vi "Durability_will_2012_07_04.vi"() -> ()   [LabVIEW 2011]
uses:
  <vilib>/DAQmx/write.llb/DAQmx Write (Counter Time 1Chan 1Samp).vi
  <vilib>/DAQmx/read.llb/DAQmx Read (Analog 1D Wfm NChan NSamp).vi
  <vilib>/express/express shared/ex_Modify Signal Name.vi
  <vilib>/measure/madcrms.llb/Basic Averaged DC-RMS for 1 Chan.vi
  <vilib>/DAQmx/miscellaneous.llb/DAQmx Fill In Error Info.vi
  <vilib>/express/express arith-compare/Formula/XNode/ExpressFormulaBlockNode.xnode
  <vilib>/measure/NI_MAPro.lvlib
  <vilib>/Analysis/NI_AALBase.lvlib
panel:
  out "Collected Signals":dynamicdata(graph)
  out "Table":string[][](table)
  in  "Filename 2":path=path "\\\\vmware-host\\Shared Folders/Desktop/long.tdms" caption="Filename"
  in  "Filename":path=path "\\\\vmware-host\\Shared Folders/Desktop/short.tdms"
  out "RPM Graph":dbl(graph)
  out "Motor RPM":dbl format="%#.0f"
  out "Motor Power (watts)":dbl format="%#.4f"
  out "Power to MC1 (watts)":dbl format="%#.4f"
  out "Voltage to MC1 (volts)":dbl format="%#.4f"
  out "Current to MC1  (amps)":dbl format="%#.4f"
  in  "Manual Start":bool
  in  "Power \nSetting":i8(slide) min=0 max=100 step=10 scale=0.0..100.0
  out "Power Setting (%)":dbl format="%#.2f"
  out "Motor Temp (F)":dbl format="%.1f"
  out "Tank Temp (F)":dbl format="%.1f"
  in  "Quit 4":bool
  out "Motor Power Over Time":dbl(graph)
  out "Phase to Phase Voltage":waveform(dbl)(graph)
  out "Phase Current":waveform(dbl)(graph)
  # "Motor Power and RPM"
  # "Temperature"
  # "MC1"
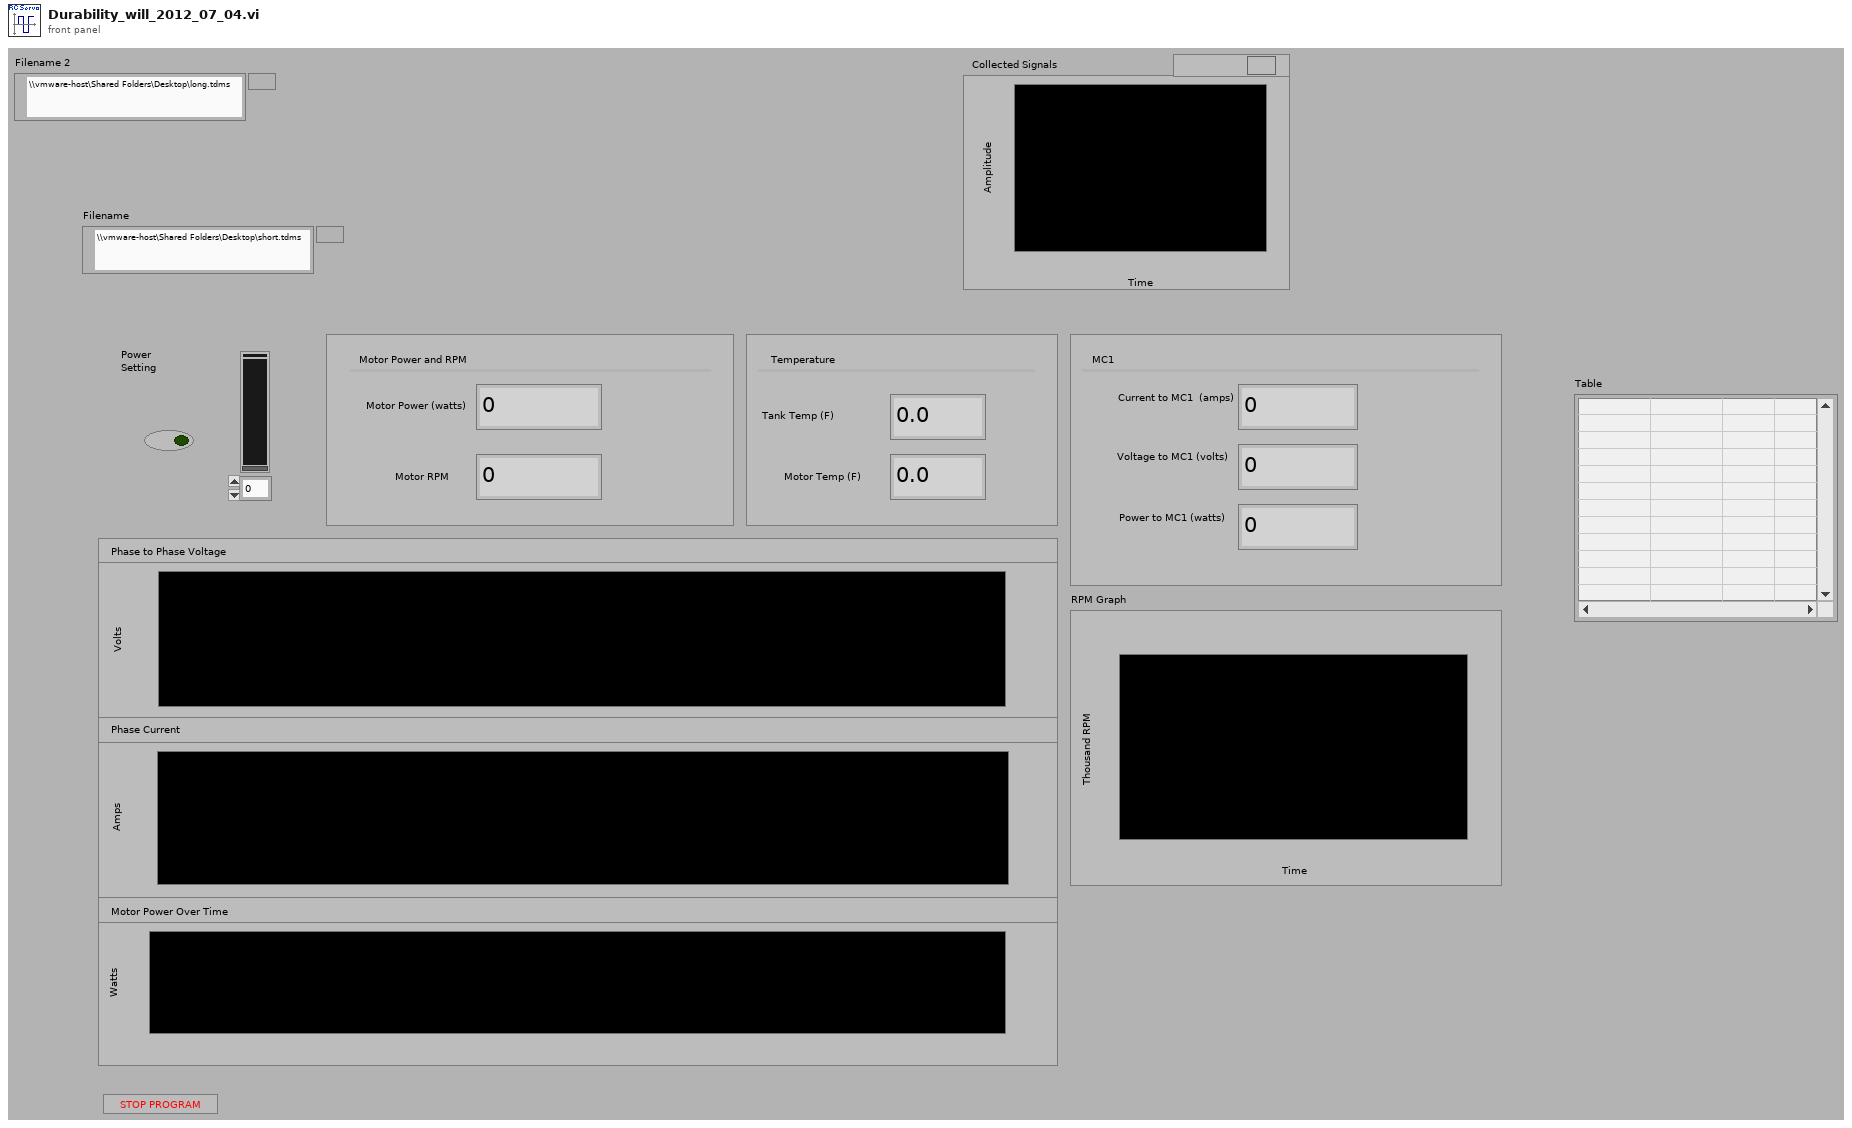
[diagram p1: front panel]
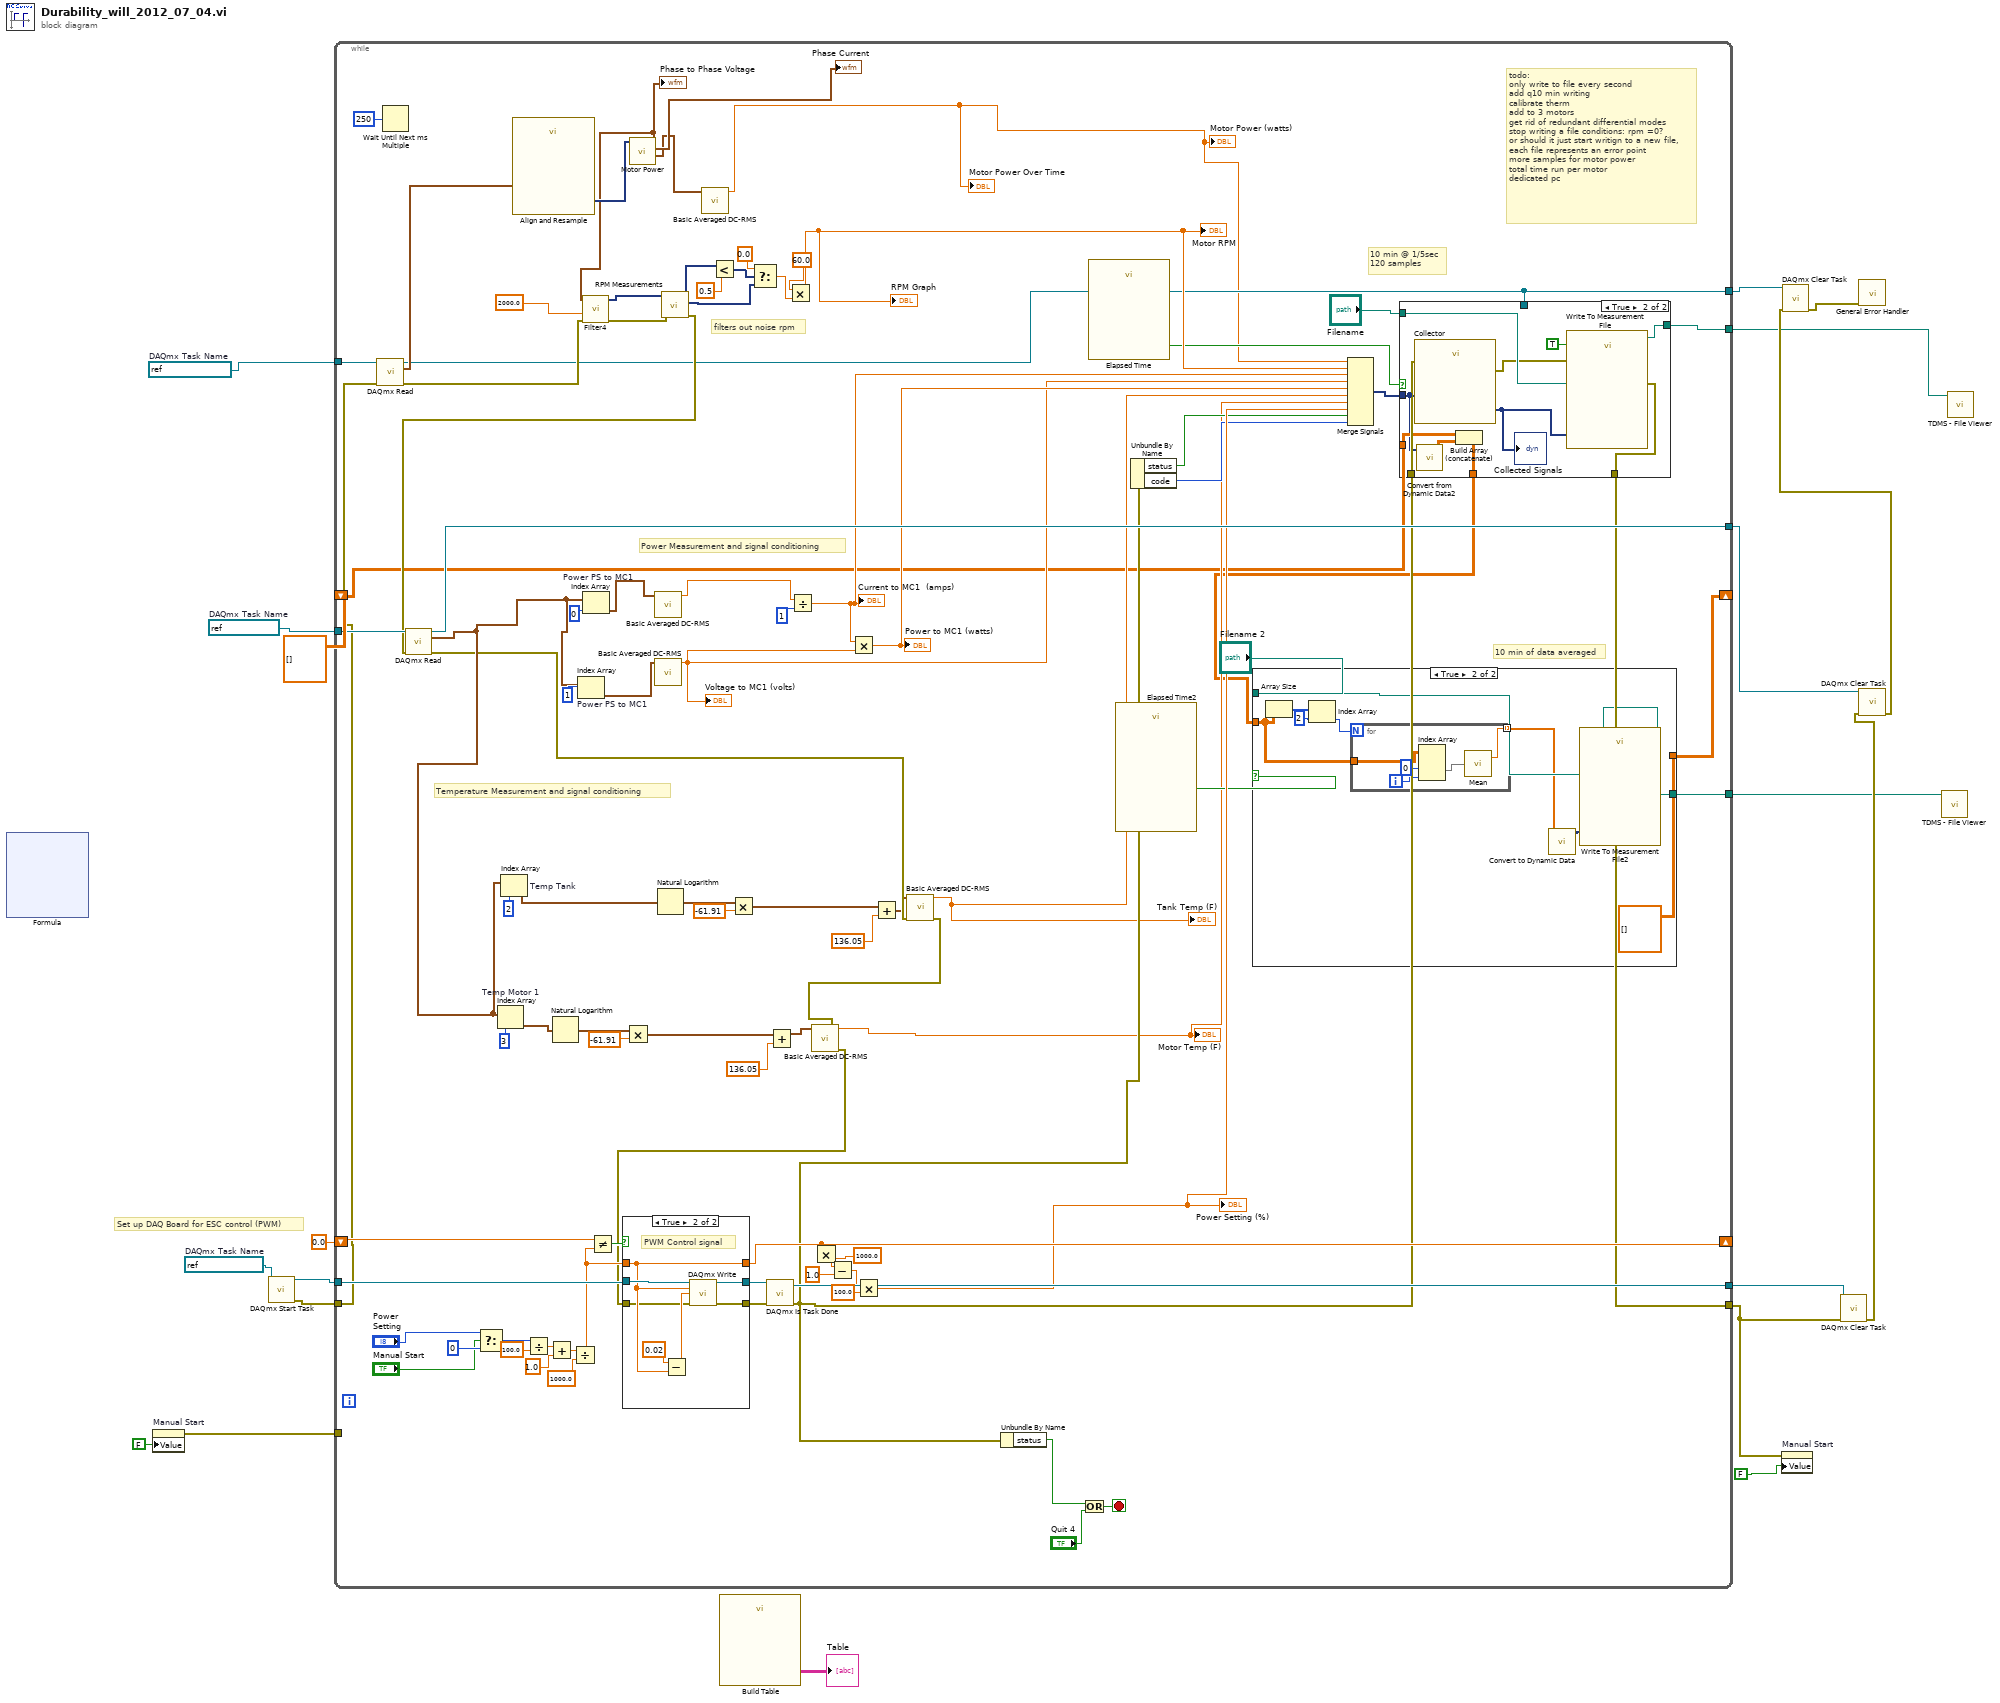
[diagram p0: block diagram]
diagram:
  w11 = refnum<k21> "PWM Signal"  # DAQmx Task Name
  w16 = refnum<k21> "MC Power"  # DAQmx Task Name
  w17 = refnum<k21> "Motor Power"  # DAQmx Task Name
  # "Set up DAQ Board for ESC control (PWM)"
  n1 = xnode "Formula"() -> ()  [unwired: 2 in, 2 out]
  n2 = property on="Manual Start" class="Bool (strict)"("Value"=FALSE ("Run Motor")) -> (error out=w14:errorcluster)  [unwired: 2 in, 1 out]
  n3 = call <vilib>:"DAQmx Start Task.vi"("task/channels in"=w11) -> ("task out"=w10:refnum<k21>, "error out"=w9:errorcluster)  [unwired: 13 in]
  n4 = while {
    tunnel: [w114] -> w20
    tunnel: [w47] -> w12
    tunnel: w10 -> [w112]
    shift-right: [w95] -> _
    shift-left: 0.0 -> [w103]
    tunnel: w16 -> [w90]
    tunnel: [w89] -> w19
    tunnel: [w46] -> w18
    tunnel: w17 -> [w76]
    tunnel: w14 -> [_]
    tunnel: w9 -> [w69]
    shift-right: [w23] -> _
    shift-left: dbl[][][] [] -> [w22]
    tunnel: [w42] -> w5
    tunnel: [w39] -> w4
    stop <- w72 stop-if-true
    # "10 min of data averaged"
    # "todo:\nonly write to file every second\nadd q10 min writing\ncalibrate therm\nadd to 3 motors\nget rid of redundant differential modes\nstop writing a file conditions: rpm =0?\nor should it just start writign to a new file,\neach file represents an error point\nmore samples for motor power\ntotal time run per motor\ndedicated pc"
    # "filters out noise rpm"
    # "10 min @ 1/5sec\n120 samples"
    # "Power Measurement and signal conditioning"
    # "Temperature Measurement and signal conditioning"
    n5 = call-poly <vilib>:"DAQmx Read.vi"("task/channels in"=w76, "error in"=w69) -> ("task out"=w46:refnum<k21>, "data"=w51:waveform(dbl)[], "error out"=w86:errorcluster)  [unwired: 11 in]
    n6 = Wait Until Next ms Multiple(millisecond multiple=u32 250) -> ()  [unwired: 1 out]
    n7 = Select(t="Power \nSetting", s="Manual Start", f=i8 0) -> (s? t:f=w101:i8)
    n8 = call "Align and Resample"("Signals"=w51) -> ("Resampled Signals"=w52:dynamicdata)  [unwired: 8 in, 2 out]
    n9 = Divide(x=w101, y=100.0) -> (x/y=w107:dbl)
    n10 = Add(x=w107, y=1.0 ("x/y")) -> (x+y=w105:dbl)
    n11 = Divide(x=w105, y=1000.0) -> (x/y=w104:dbl)
    n12 = Not Equal?(x=w103, y=w104) -> (x != y?=w113:bool)
    n13 = call "Motor Power.vi"("data"=w52) -> ("Waveform"=w38:waveform(dbl), "Phase Current"=→"Phase Current":waveform(dbl), "Phase to Phase Voltage"=w49:waveform(dbl))  [unwired: 7 in, 1 out]
    "Phase to Phase Voltage" <- w49
    n14 = call "Filter4"("error in (no error)"=w86, "Lower Cut-Off"=2000.0 ("LowPass Filter CutOff [Hz]"), "Signal"=w49) -> ("error out"=w87:errorcluster, "Filtered Signal"=w78:dynamicdata)  [unwired: 7 in]
    n15 = call "RPM Measurements"("error in (no error)"=w87, "Signals"=w78) -> ("error out"=w71:errorcluster, "Frequency"=w82:dynamicdata, "Amplitude"=w79:dynamicdata)  [unwired: 7 in]
    n16 = call-poly <vilib>:"DAQmx Read.vi"("task/channels in"=w90, "error in"=w71) -> ("task out"=w89:refnum<k21>, "data"=w31:waveform(dbl)[], "error out"=w29:errorcluster)  [unwired: 11 in]
    n17 = Index Array "Temp Motor 1"(array=w31, index=3) -> (element=w64:waveform(dbl))
    n18 = Index Array "Temp Tank"(array=w31, index=2) -> (element=w32:waveform(dbl))
    n19 = Natural Logarithm(1:w64) -> (0:w68:waveform(dbl))
    n20 = Index Array "Power PS to MC1"(array=w31, index=1) -> (element=w34:waveform(dbl))
    n21 = Index Array "Power PS to MC1"(array=w31, index=0) -> (element=w36:waveform(dbl))
    n22 = Multiply(x=w68, y=-61.91) -> (x*y=w66:waveform(dbl))
    n23 = call-poly <vilib>:"Basic Averaged DC-RMS.vi"("signal in"=w36) -> ("DC value"=w35:dbl)  [unwired: 7 in, 3 out]
    n24 = call-poly <vilib>:"Basic Averaged DC-RMS.vi"("signal in"=w34) -> ("DC value"=w33:dbl)  [unwired: 7 in, 3 out]
    "Voltage to MC1 (volts)" <- w33
    n25 = Natural Logarithm(1:w32) -> (0:w63:waveform(dbl))
    n26 = call-poly <vilib>:"Basic Averaged DC-RMS.vi"("signal in"=w38) -> ("DC value"=w37:dbl)  [unwired: 7 in, 3 out]
    "Motor Power Over Time" <- w37
    "Motor Power (watts)" <- w37
    n27 = Less?(x=w79, y=0.5) -> (x < y?=w81:dynamicdata)
    n28 = Multiply(x=w63, y=-61.91) -> (x*y=w61:waveform(dbl))
    n29 = Select(t=0.0, s=w81, f=w82) -> (s? t:f=w84:dbl)
    n30 = Add(x=w66, y=136.05) -> (x+y=w27:waveform(dbl))
    n31 = Multiply(x=60.0, y=w84) -> (x*y=w58:dbl)
    "Motor RPM" <- w58
    "RPM Graph" <- w58
    n32 = Divide(x=w35, y=1) -> (x/y=w57:dbl)
    "Current to MC1  (amps)" <- w57
    n33 = Multiply(x=w57, y=w33) -> (x*y=w56:dbl)
    "Power to MC1 (watts)" <- w56
    n34 = Add(x=w61, y=136.05) -> (x+y=w28:waveform(dbl))
    n35 = call-poly <vilib>:"Basic Averaged DC-RMS.vi"("error in (no error)"=w29, "signal in"=w28) -> ("error out"=w24:errorcluster, "DC value"=w30:dbl)  [unwired: 6 in, 2 out]
    "Tank Temp (F)" <- w30
    n36 = call-poly <vilib>:"Basic Averaged DC-RMS.vi"("error in (no error)"=w24, "signal in"=w27) -> ("error out"=w25:errorcluster, "DC value"=w26:dbl)  [unwired: 6 in, 2 out]
    "Motor Temp (F)" <- w26
    n37 = case shown="True" w113 {
      tunnel: w104 -> [w146 w149]
      tunnel: w112 -> [w147 w153]
      tunnel: [w147 w151] -> w111
      tunnel: [w145 w150] -> w110
      tunnel: [w146 w149] -> w95
      tunnel: w25 -> [w145 w148]
      frame False {
      }
      frame True {
        # "PWM Control signal"
        n38 = Subtract(x=0.02, y=w149) -> (x-y=w152:dbl)
        n39 = call-poly <vilib>:"DAQmx Write.vi"("task/channels in"=w153, "high time"=w149, "low time"=w152, "error in"=w148) -> ("task out"=w151:refnum<k21>, "error out"=w150:errorcluster)  [unwired: 9 in, 1 out]
      }
    }
    n40 = call <vilib>:"DAQmx Is Task Done.vi"("task/channels in"=w111, "error in"=w110) -> ("task out"=w114:refnum<k21>, "error out"=w48:errorcluster)  [unwired: 11 in, 1 out]
    n41 = Multiply(x=w95, y=1000.0) -> (x*y=w96:dbl)
    n42 = Subtract(x=w96, y=1.0) -> (x-y=w99:dbl)
    n43 = Multiply(x=w99, y=100.0) -> (x*y=w55:dbl)
    "Power Setting (%)" <- w55
    n44 = Unbundle By Name(w48) -> ("status"=w70:bool)
    n45 = Or(x=w70, y="Quit 4") -> (x .or. y?=w72:bool)
    n46 = call "Elapsed Time"() -> ("Time has Elapsed"=w45:bool)  [unwired: 12 in, 7 out]
    n47 = call "Elapsed Time2"() -> ("Time has Elapsed"=w44:bool)  [unwired: 12 in, 7 out]
    n48 = Unbundle By Name(w48) -> ("status"=w54:bool, "code"=w53:i32)
    n49 = Merge Signals(w37, w58, w57, w33, w56, w30, w26, w55, w54, w53) -> (w43:dynamicdata)
    n50 = case shown="True" w45 {
      tunnel: w43 -> [_ w135]
      tunnel: w48 -> [w133 w144]
      tunnel: [w133 w141] -> w47
      tunnel: w46 -> [_ _]
      tunnel: "Filename" -> [w132 w143]
      tunnel: [w132 w140] -> w39
      tunnel: [w131 w137] -> w21
      tunnel: w22 -> [w131 w136]
      frame False {
      }
      frame True {
        n51 = call "Collector"("error in (no error)"=w144, "Signals"=w135) -> ("error out"=w142:errorcluster, "Collected Signals"=w139:dynamicdata)  [unwired: 8 in]
        "Collected Signals" <- w139
        n52 = call "Convert from Dynamic Data2"("Dynamic Data Type"=w135) -> ("Array"=w134:dbl[][])  [unwired: 3 in]
        n53 = Build Array (concatenate)(w136, w134) -> (w137:dbl[][][])
        n54 = call "Write To Measurement File"("Signals"=w139, "Reset"=TRUE, "error in (no error)"=w142, "Filename"=w143) -> ("Filename Out"=w140:path, "error out"=w141:errorcluster)  [unwired: 13 in, 1 out]
      }
    }
    n55 = case shown="True" w44 {
      tunnel: w21 -> [w115 w122]
      tunnel: [w116 w125] -> w42
      tunnel: "Filename 2" -> [w116 w124]
      tunnel: [w115 dbl[][][] []] -> w23
      frame False {
      }
      frame True {
        n56 = Array Size(array=w122) -> (size(s)=w118:i32[])
        n57 = Index Array(array=w118, index=2) -> (element=w119:i32)
        n58 = for {
          N: w119 -> [_]
          tunnel: w122 -> [w130]
          tunnel: [w126] -> w117 mode=indexing
          i -> [w129]
          n59 = Index Array(array=w130, index (dim 1)=0 ("disabled index (row)"), index (dim 2)=w129) -> (element=w128:dbl[])  [unwired: 1 in]
          n60 = call <vilib>:"Mean.vi"("X"=w128) -> ("mean"=w126:dbl)  [unwired: 1 out]
        }
        n61 = call "Convert to Dynamic Data"("Array"=w117) -> ("Dynamic Data Type"=w123:dynamicdata)  [unwired: 3 in]
        n62 = call "Write To Measurement File2"("Signals"=w123, "Filename"=w124) -> ("Filename Out"=w125:path)  [unwired: 15 in, 2 out]
      }
    }
  }
  n63 = call "Build Table"() -> ("Table"=→"Table":string[][])  [unwired: 5 in, 6 out]
  n64 = property on="Manual Start" class="Bool (strict)"(error in=w12, "Value"=FALSE ("Run Motor")) -> ()  [unwired: 1 in, 2 out]
  n65 = call <vilib>:"DAQmx Clear Task.vi"("task in"=w20, "error in"=w12) -> ("error out"=w6:errorcluster)  [unwired: 13 in]
  n66 = call <vilib>:"DAQmx Clear Task.vi"("task in"=w19, "error in"=w6) -> ("error out"=w8:errorcluster)  [unwired: 13 in]
  n67 = call <vilib>:"DAQmx Clear Task.vi"("task in"=w18, "error in"=w8) -> ("error out"=w7:errorcluster)  [unwired: 13 in]
  n68 = call <vilib>:"General Error Handler.vi"("error in (no error)"=w7) -> ()  [unwired: 10 in, 5 out]
  n69 = call <vilib>:"TDMS - File Viewer.vi"("file path"=w5) -> ()  [unwired: 1 in, 6 out]
  n70 = call <vilib>:"TDMS - File Viewer.vi"("file path"=w4) -> ()  [unwired: 1 in, 6 out]
